vi "Set Robot Virtual Mode.vi"(8 "error in":errorcluster, 11 "Gantry in":refnum<class "Gantry Class.lvclass">) -> (0 "error out":errorcluster, 3 "Gantry out":refnum<class "Gantry Class.lvclass">)   [LabVIEW 2017, in "Gantry Class.lvclass"]
uses:
  Gantry Class.lvclass
  Gantry Class.lvclass/Gantry Class.ctl
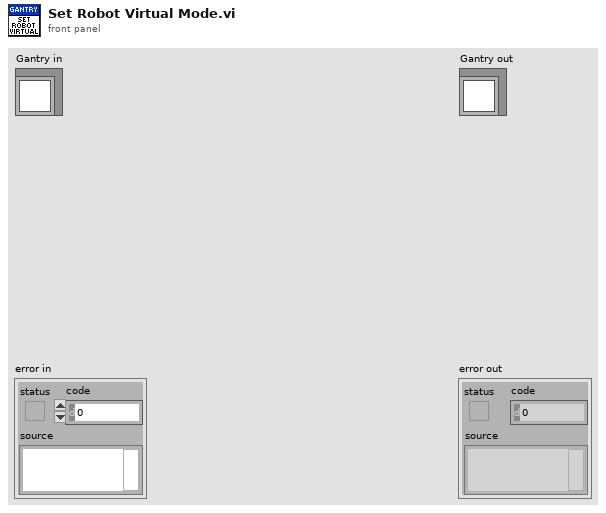
[diagram p1: front panel]
types:
  T1 = typedef "Virtual Modes.ctl" = enum16{"Nonvirtual", "Pseudovirtual", "Virtual"}
  T2 = typedef "ControllerDiagPacket.ctl" = cluster{"Number of Diag Packets":i32, "Axes":T3[], "error":errorcluster}
  T3 = typedef "AxisDiagPacket.ctl" = cluster{"Axis Name":string, "Analog Input 0":dbl, "Analog Input 1":dbl, "Axis Fault (num)":i32, "Axis Fault (str)":string, "Axis Fault (bits)":cluster{"AmplifierFault":bool, "AmplifierTemperatureFault":bool, "CcwEndOfTravelLimitFault":bool, "CcwSoftwareLimitFault":bool, "CommunicationLostFault":bool, "CwEndOfTravelLimitFault":bool, "CwSoftwareLimitFault":bool, "EmergencyStopFault":bool, "EncoderFault":bool, "ExternalFault":bool, "FeedbackScalingFault":bool, "GantryMisalignFault ":bool, "HallSensorFault":bool, "InPositionTimeout":bool, "MarkerSearchFault":bool, "MaxVelocityCommandFault":bool, "MotorTemperatureFault":bool, "None":bool, "OverCurrentFault":bool, "PositionErrorFault":bool, "PositionFeedbackFault":bool, "ProbeInputFault":bool, "SafeZoneFault":bool, "VelocityErrorFault":bool, "VelocityFeedbackFault":bool}, "Axis Status (num)":i32, "Axis Status (str)":string, "Axis Status (bits)":cluster{"BacklashActive":bool, "CalibrationEnabled1D":bool, "CalibrationEnabled2D":bool, "CommandValid":bool, "DrivePending":bool, "Enabling":bool, "GainCalibrationEnabled":bool, "GantryAligned":bool, "GantryRealigning":bool, "Homed":bool, "Homing":bool, "Jogging":bool, "JoystickControl":bool, "MasterSlaveControl":bool, "MotionBlocked":bool, "MotionClamped":bool, "MoveDone":bool, "None":bool, "NotVirtual":bool, "Profiling":bool, "Stability0":bool, "Stability1":bool, "TrajectoryFiltering":bool, "WaitDone":bool}, "Current Command":sgl, "Current Error":sgl, "Current Feedback":sgl, "Digital Inputs":i32, "Digital Outputs":i32, "Drive Status":i32, "Drive Status (str)":string, "Drive Status (bits)":cluster{"AccelerationPhase":bool, "AutofocusActive":bool, "BrakeOutput":bool, "CcwEndOfTravelLimitInput":bool, "CosineEncoderError":bool, "CurrentClamp":bool, "CwEndOfTravelLimitInput":bool, "DecelerationPhase":bool, "DualLoopActive":bool, "EmergencyStopInput":bool, "Enabled":bool, "EncoderClipping":bool, "GalvoFifoFull":bool, "GalvoSubMsecMode":bool, "HallAInput":bool, "HallBInput":bool, "HallCInput":bool, "HighResolutionMode":bool, "HomeLimitInput":bool, "InPosition":bool, "MarkerInput":bool, "MarkerLatch":bool, "MoveActive":bool, "NoMotorSupply":bool, "None":bool, "PowerLimiting":bool, "ProgrammingFlash":bool, "ProgrammingMXH":bool, "PSOHaltLatch":bool, "SineEncoderError":bool}, "Position Feedback Auxiliary":dbl, "Position Command":dbl, "Position Error":dbl, "Position Feedback":dbl, "Program Position Command":dbl, "Program Position Error":dbl, "Program Position Feedback":dbl, "Velocity Command":dbl, "Velocity Error":dbl, "Velocity Feedback":dbl}
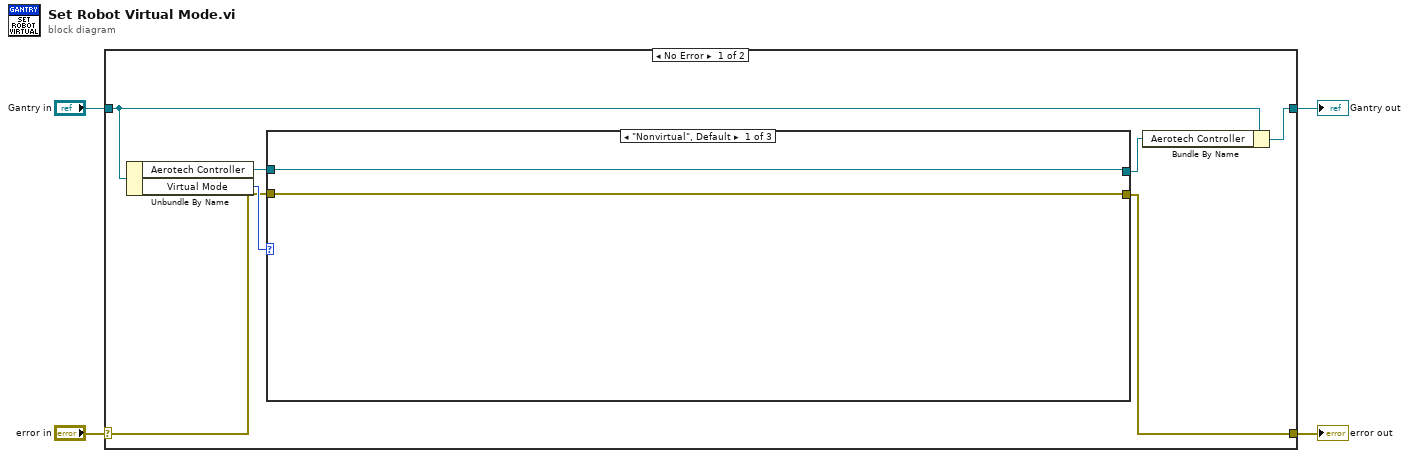
[diagram p0: block diagram]
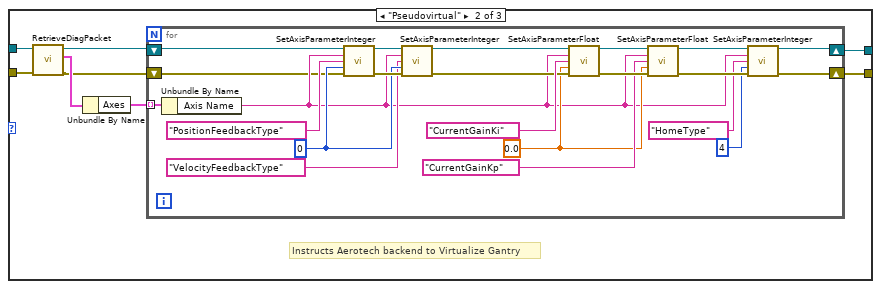
[diagram p2: hidden frame]
diagram:
  n1 = case shown="No Error" "error in" {
    selector: "error in" -> [w6 w47]
    tunnel: [w5 w47] -> w3
    tunnel: [w8 w46] -> w1
    tunnel: "Gantry in" -> [w9 w46]
    frame No Error {
      n2 = Unbundle By Name(w9) -> ("Aerotech Controller"=w10:refnum<k24>, "Virtual Mode"=w11:T1)
      n3 = case shown="\"Nonvirtual\", Default" w11 {
        tunnel: w10 -> [w13 w21 w45]
        tunnel: [w13 w17 w45] -> w7
        tunnel: w6 -> [w12 w16 w44]
        tunnel: [w12 w14 w44] -> w5
        frame "Nonvirtual", Default {
        }
        frame "Pseudovirtual" {
          # "Instructs Aerotech backend to Virtualize Gantry"
          n4 = call <userlib>:"RetrieveDiagPacket.vi"("error in (no error)"=w16, "Controller In"=w21) -> ("error out"=w15:errorcluster, "ControllerDiagPacket"=w19:T2, "Controller Out"=w20:refnum<k24>)  [unwired: 7 in]
          n5 = Unbundle By Name(w19) -> ("Axes"=w18:T3[])
          n6 = for {
            tunnel: w18 -> [w42] mode=indexing
            shift-right: [w24] -> w17
            shift-left: w20 -> [w43]
            shift-right: [w22] -> w14
            shift-left: w15 -> [w23]
            w30 = sgl 0.0 ("value")
            w38 = 0 ("value")
            n7 = Unbundle By Name(w42) -> ("Axis Name"=w27:string)
            n8 = call <userlib>:"SetAxisParameterInteger.vi"("Controller In"=w43, "axisName"=w27, "Parameter Name"="PositionFeedbackType", "value"=w38, "error in (no error)"=w23) -> ("Controller Out"=w40:refnum<k24>, "error out"=w39:errorcluster)  [unwired: 9 in]
            n9 = call <userlib>:"SetAxisParameterInteger.vi"("Controller In"=w40, "axisName"=w27, "Parameter Name"="VelocityFeedbackType", "value"=w38, "error in (no error)"=w39) -> ("Controller Out"=w36:refnum<k24>, "error out"=w32:errorcluster)  [unwired: 9 in]
            n10 = call <userlib>:"SetAxisParameterFloat.vi"("Controller In"=w36, "axisName"=w27, "Parameter Name"="CurrentGainKi", "value"=w30, "error in (no error)"=w32) -> ("Controller Out"=w34:refnum<k24>, "error out"=w33:errorcluster)  [unwired: 9 in]
            n11 = call <userlib>:"SetAxisParameterFloat.vi"("Controller In"=w34, "axisName"=w27, "Parameter Name"="CurrentGainKp", "value"=w30, "error in (no error)"=w33) -> ("Controller Out"=w29:refnum<k24>, "error out"=w28:errorcluster)  [unwired: 9 in]
            n12 = call <userlib>:"SetAxisParameterInteger.vi"("Controller In"=w29, "axisName"=w27, "Parameter Name"="HomeType", "value"=4, "error in (no error)"=w28) -> ("Controller Out"=w24:refnum<k24>, "error out"=w22:errorcluster)  [unwired: 9 in]
          }
        }
        frame "Virtual" {
          # "Bypass Aerotech VI's completely"
        }
      }
      n13 = Bundle By Name(cluster=w9, "Aerotech Controller"=w7) -> (w8:refnum<class "Gantry Class.lvclass">)
    }
    frame Error {
    }
  }
  "error out" <- w3
  "Gantry out" <- w1
